vi "Get All Property Names.vi"(8 "error in":errorcluster, 11 "Item Ref in":refnum<data-value>) -> (0 "error out":errorcluster, 3 "Property Names":string[](array[string]))   [LabVIEW 2024, in "Config File Parser.lvlib" / "Property.lvclass"]
uses:
  Property.lvclass
  Item/Item.lvclass
  Property.lvclass/Property.ctl
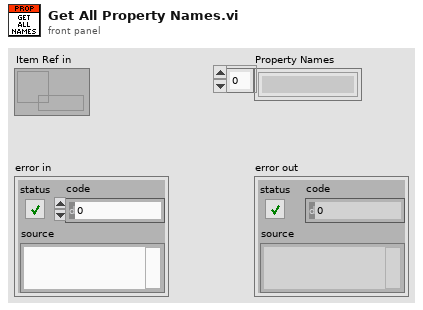
[diagram p1: front panel]
types:
  T1 = typedef "Config File Parser.lvlib/Item.lvclass/Item Type.ctl" = enum16{"Property", "Channel", "Section"}
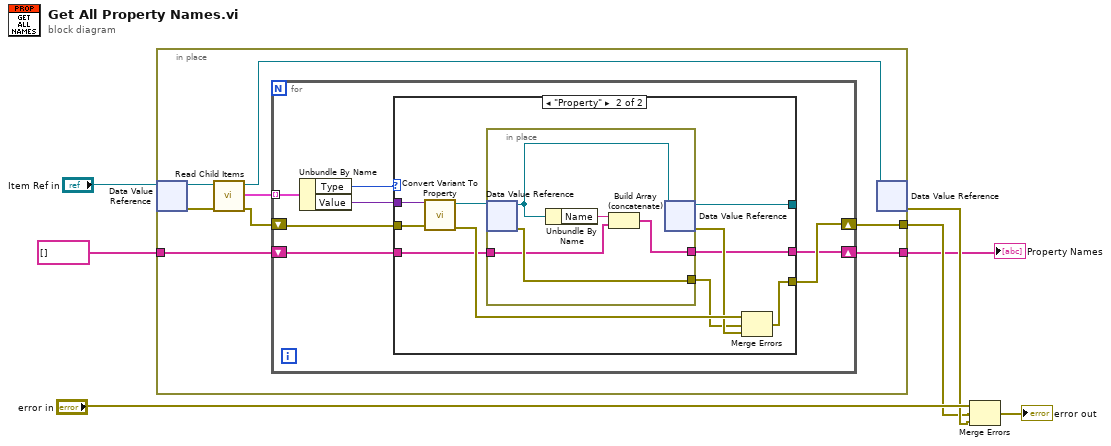
[diagram p0: block diagram]
diagram:
  n1 = in-place {
    in-place-border: string[] [] -> [w10]
    in-place-border: [w13] -> w4
    in-place-border: [w9] -> w1
    n2 = in-place-dvr #1("Item Ref in") -> (w12:refnum<class "Item.lvclass">, w15:errorcluster)
    n3 = call-dynamic "Read Child Items.vi"("error in"=w15, "Item in"=w12) -> ("error out"=w14:errorcluster, "Child Items"=w11:cluster{"Type":T1, "Value":variant}[], "Item out"=w8:refnum<class "Item.lvclass">)  [unwired: 7 in]
    n4 = for {
      tunnel: w11 -> [w20] mode=indexing
      shift-right: [w21] -> w13
      shift-left: w14 -> [w22]
      shift-right: [w16] -> w9
      shift-left: w10 -> [w17]
      n5 = Unbundle By Name(w20) -> ("Type"=w19:T1, "Value"=w18:variant)
      n6 = case shown="\"Property\"" w19 {
        tunnel: w18 -> [_ w29]
        tunnel: [_ w27] -> _
        tunnel: w22 -> [w24 w34]
        tunnel: [w24 w31] -> w21
        tunnel: w17 -> [w23 w26]
        tunnel: [w23 w25] -> w16
        frame Default {
        }
        frame "Property" {
          n7 = call "Convert Variant To Property.vi"("error in"=w34, "Property Variant"=w29) -> ("error out"=w33:errorcluster, "Property Ref out"=w28:refnum<data-value>)  [unwired: 8 in]
          n8 = in-place {
            in-place-border: w26 -> [w37]
            in-place-border: [w36] -> w25
            in-place-border: [w39] -> w30
            n9 = in-place-dvr #2(w28) -> (w35:refnum<class "Property.lvclass">, w39:errorcluster)
            n10 = Unbundle By Name(w35) -> ("Name"=w38:string)
            n11 = Build Array (concatenate)(w38, w37) -> (w36:string[])
            n12 = in-place-dvr #2(w35) -> (w27:refnum<data-value>, w32:errorcluster)
          }
          n13 = Merge Errors(w33, w30, w32) -> (w31:errorcluster)
        }
      }
    }
    n14 = in-place-dvr #1(w8) -> (w6:errorcluster)  [unwired: 1 out]
  }
  "Property Names" <- w1
  n15 = Merge Errors("error in", w4, w6) -> (→"error out":errorcluster)
